vi "RichToFlatnixnet_grpc_FutureTimeTriggerRequest.vi"(5 "OutputClusterType":T1, 11 "InputCluster":T4) -> (3 "OutputCluster":T1)   [LabVIEW 2025, in "xnet-grpc_client.lvlib"]
uses:
  xnet-grpc_client.lvlib
  nixnet_grpc_FutureTimeTriggerRequest.ctl
  nixnet_grpc_FutureTimeTriggerRequest_timescale_enum/nixnet_grpc_FutureTimeTriggerRequest_timescale_enum.lvclass
  nidevice_grpc_Session.ctl
  nixnet_grpc_FutureTimeTriggerRequest_Flat.ctl
  nidevice_grpc_Session_Flat.ctl
  nixnet_grpc_TimeScale.ctl
  nixnet_grpc_FutureTimeTriggerRequest_timescale_enum/nixnet_grpc_FutureTimeTriggerRequest_timescale_enum.lvclass/nixnet_grpc_FutureTimeTriggerRequest_timescale_enum.ctl
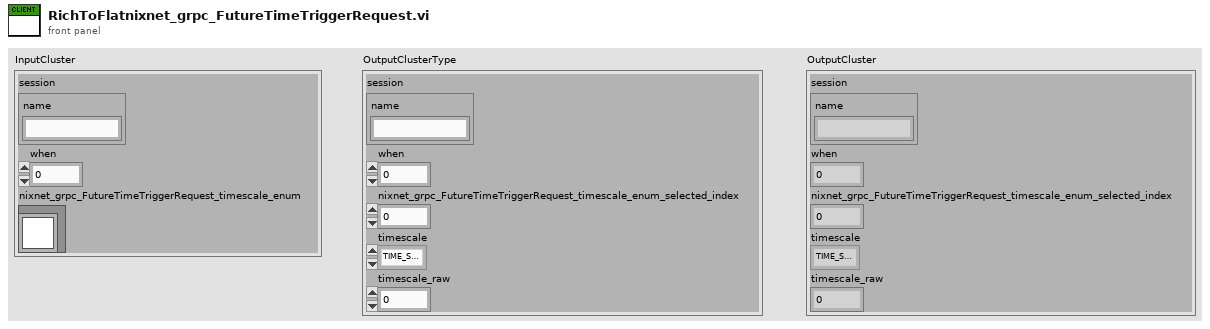
[diagram p1: front panel]
types:
  T1 = typedef "xnet-grpc_client.lvlib/nixnet_grpc_FutureTimeTriggerRequest_Flat.ctl" = cluster{"session":T2, "when":u64, "nixnet_grpc_FutureTimeTriggerRequest_timescale_enum_selected_index":i32, "timescale":T3, "timescale_raw":u32}
  T2 = typedef "xnet-grpc_client.lvlib/nidevice_grpc_Session_Flat.ctl" = cluster{"name":string}
  T3 = typedef "xnet-grpc_client.lvlib/nixnet_grpc_TimeScale.ctl" = enum32{"TIME_SCALE_LOCAL_TIME", "TIME_SCALE_NETWORK_TIME"}
  T4 = typedef "xnet-grpc_client.lvlib/nixnet_grpc_FutureTimeTriggerRequest.ctl" = cluster{"session":T5, "when":u64, "nixnet_grpc_FutureTimeTriggerRequest_timescale_enum":refnum<class "nixnet_grpc_FutureTimeTriggerRequest_timescale_enum.lvclass">}
  T5 = typedef "xnet-grpc_client.lvlib/nidevice_grpc_Session.ctl" = cluster{"name":string}
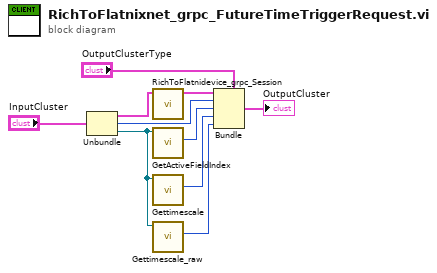
[diagram p0: block diagram]
diagram:
  n1 = Unbundle "Unbundle"("InputCluster") -> ("session"=w7:T5, "when"=w5:u64, "nixnet_grpc_FutureTimeTriggerRequest_timescale_enum"=w4:refnum<class "nixnet_grpc_FutureTimeTriggerRequest_timescale_enum.lvclass">)
  n2 = call "RichToFlatnidevice_grpc_Session.vi"("InputCluster"=w7) -> ("OutputCluster"=w6:T2)  [unwired: 10 in]
  n3 = call "GetActiveFieldIndex.vi"("OneOfTemplate in"=w4) -> ("Active Field Index"=w3:i32)  [unwired: 8 in, 2 out]
  n4 = call "Gettimescale.vi"("OneOfTemplate in"=w4) -> ("Get_Val"=w2:T3)  [unwired: 8 in, 2 out]
  n5 = call "Gettimescale_raw.vi"("OneOfTemplate in"=w4) -> ("Get_Val"=w1:u32)  [unwired: 8 in, 2 out]
  n6 = Bundle "Bundle"(cluster="OutputClusterType", "session"=w6, "when"=w5, "nixnet_grpc_FutureTimeTriggerRequest_timescale_enum_selected_index"=w3, "timescale"=w2, "timescale_raw"=w1) -> (→"OutputCluster":T1)
